vi "myRIO__TCP_constants_byteRange_letters.vi"() -> (0 "output_byte_end_uppercase":u8=90, 1 "output_byte_end_lowercase":u8=122, 2 "output_byte_start_uppercase":u8=65, 3 "output_byte_start_lowercase":u8=97)   [LabVIEW 2014]
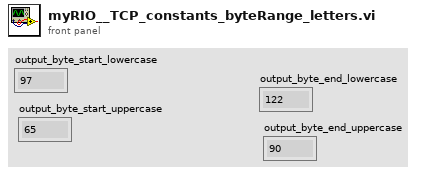
[diagram p1: front panel]
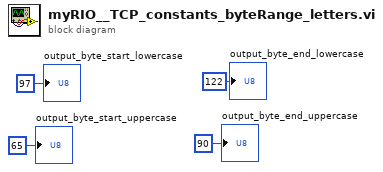
[diagram p0: block diagram]
diagram:
  "output_byte_end_lowercase" <- u8 122
  "output_byte_end_uppercase" <- u8 90
  "output_byte_start_lowercase" <- u8 97
  "output_byte_start_uppercase" <- u8 65
